vi "Set Security Level CORE.vi"(8 "error in (no error)":errorcluster, 9 "Set or Clear":T1, 10 "New Level":T2, 11 "Threat Deterent in":refnum<class "Threat Deterent.lvclass">) -> (0 "error out":errorcluster, 2 "Last Action Performed":string, 3 "Threat Deterent out":refnum<class "Threat Deterent.lvclass">)   [LabVIEW 2014, in "Threat Deterent.lvclass"]
uses:
  Threat Deterent.lvclass
  Security System/Security Level.ctl
  Security System/Set or Clear.ctl
  Threat Deterent.lvclass/Threat Deterent.ctl
  Electric Fence/Electric Fence.lvclass
  Security System/Security System.lvclass
  Rabbit Squad/Rabbit Squad.lvclass
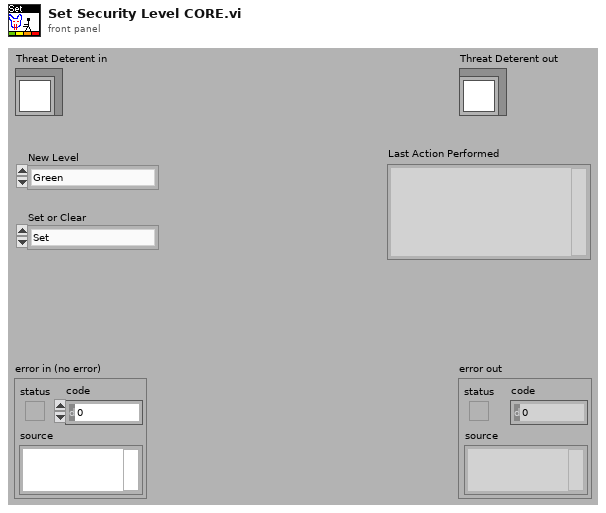
[diagram p1: front panel]
types:
  T1 = typedef "Security System.lvclass/Set or Clear.ctl" = enum16{"Set", "Clear"}
  T2 = typedef "Security System.lvclass/Security Level.ctl" = enum16{"Green", "Yellow", "Orange", "Red"}
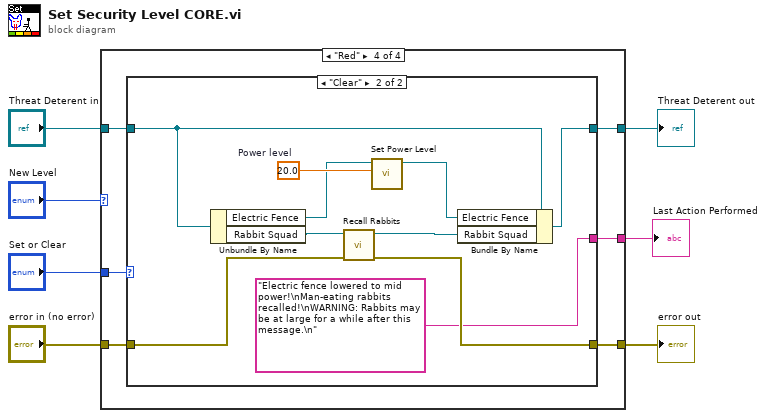
[diagram p0: block diagram]
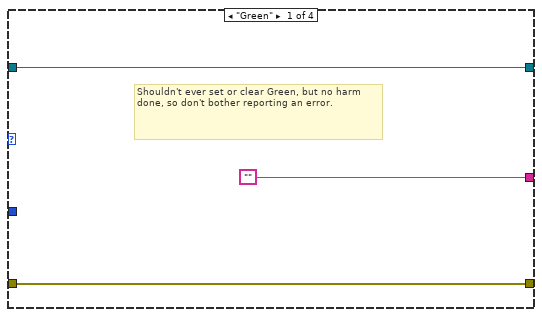
[diagram p2: hidden frame]
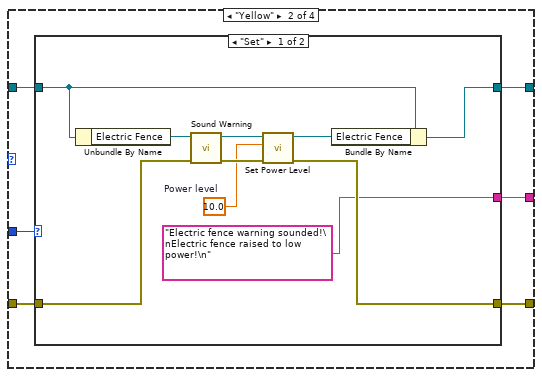
[diagram p3: hidden frame]
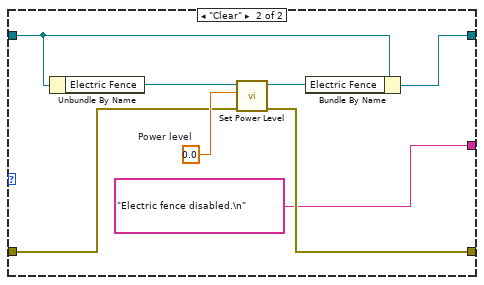
[diagram p4: hidden frame]
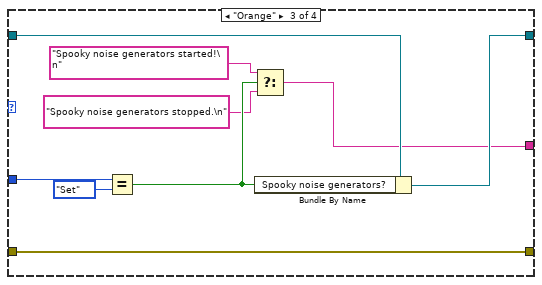
[diagram p5: hidden frame]
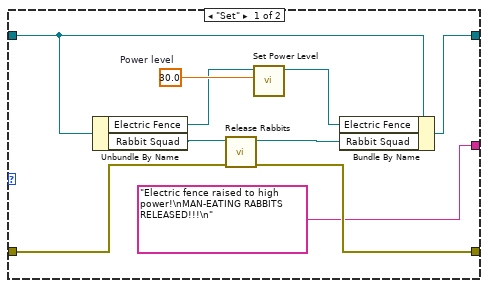
[diagram p6: hidden frame]
diagram:
  n1 = case shown="\"Red\"" "New Level" {
    tunnel: [w9 w12 w40 w45] -> w2
    tunnel: "Threat Deterent in" -> [w9 w13 w39 w46]
    tunnel: [w10 w15 w43 w48] -> w5
    tunnel: "error in (no error)" -> [w10 w14 w43 w47]
    tunnel: "Set or Clear" -> [_ w16 w42 w49]
    tunnel: ["" w11 w35 w44] -> w1
    frame "Green" {
      # "Shouldn't ever set or clear Green, but no harm done, so don't bother reporting an error."
    }
    frame "Yellow" {
      n2 = case shown="\"Set\"" w16 {
        tunnel: [w18 w28] -> w15
        tunnel: w14 -> [w19 w29]
        tunnel: w13 -> [w21 w32]
        tunnel: [w20 w31] -> w12
        tunnel: ["Electric fence warning sounded!\nElectric fence raised to low power!\n" ("Last Action Performed") "Electric fence disabled.\n" ("Last Action Performed")] -> w11
        frame "Set" {
          w23 = 10.0  # Power level
          n3 = Unbundle By Name(w21) -> ("Electric Fence"=w26:refnum<class "Electric Fence.lvclass">)
          n4 = call "Sound Warning.vi"("error in (no error)"=w19, "Electric Fence in"=w26) -> ("error out"=w24:errorcluster, "Electric Fence out"=w25:refnum<class "Electric Fence.lvclass">)  [unwired: 8 in]
          n5 = call "Set Power Level.vi"("error in (no error)"=w24, "Power level"=w23, "Electric Fence.lvclass in"=w25) -> ("error out"=w18:errorcluster, "Electric Fence.lvclass out"=w22:refnum<class "Electric Fence.lvclass">)  [unwired: 7 in]
          n6 = Bundle By Name(cluster=w21, "Electric Fence"=w22) -> (w20:refnum<class "Threat Deterent.lvclass">)
        }
        frame "Clear" {
          w34 = 0.0  # Power level
          n7 = Unbundle By Name(w32) -> ("Electric Fence"=w30:refnum<class "Electric Fence.lvclass">)
          n8 = call "Set Power Level.vi"("error in (no error)"=w29, "Power level"=w34, "Electric Fence.lvclass in"=w30) -> ("error out"=w28:errorcluster, "Electric Fence.lvclass out"=w33:refnum<class "Electric Fence.lvclass">)  [unwired: 7 in]
          n9 = Bundle By Name(cluster=w32, "Electric Fence"=w33) -> (w31:refnum<class "Threat Deterent.lvclass">)
        }
      }
    }
    frame "Orange" {
      n10 = Equal?(x=w42, y=Set_or_Clear."Set") -> (x = y?=w38:bool)
      n11 = Select(t="Spooky noise generators started!\n", s=w38, f="Spooky noise generators stopped.\n") -> (s? t:f=w35:string)
      n12 = Bundle By Name(cluster=w39, "Spooky noise generators?"=w38) -> (w40:refnum<class "Threat Deterent.lvclass">)
    }
    frame "Red" {
      n13 = case shown="\"Clear\"" w49 {
        tunnel: [w57 w67] -> w48
        tunnel: w47 -> [w58 w68]
        tunnel: w46 -> [w56 w66]
        tunnel: [w55 w65] -> w45
        tunnel: ["Electric fence raised to high power!\nMAN-EATING RABBITS RELEASED!!!\n" ("Last Action Performed") "Electric fence lowered to mid power!\nMan-eating rabbits recalled!\nWARNING: Rabbits may be at large for a while after this message.\n" ("Last Action Performed")] -> w44
        frame "Set" {
          w53 = 30.0  # Power level
          n14 = Unbundle By Name(w56) -> ("Electric Fence"=w52:refnum<class "Electric Fence.lvclass">, "Rabbit Squad"=w59:refnum<class "Rabbit Squad.lvclass">)
          n15 = call "Release Rabbits.vi"("error in (no error)"=w58, "Rabbit Squad in"=w59) -> ("error out"=w57:errorcluster, "Rabbit Squad out"=w54:refnum<class "Rabbit Squad.lvclass">)  [unwired: 8 in]
          n16 = call "Set Power Level.vi"("Power level"=w53, "Electric Fence.lvclass in"=w52) -> ("Electric Fence.lvclass out"=w51:refnum<class "Electric Fence.lvclass">)  [unwired: 8 in, 1 out]
          n17 = Bundle By Name(cluster=w56, "Electric Fence"=w51, "Rabbit Squad"=w54) -> (w55:refnum<class "Threat Deterent.lvclass">)
        }
        frame "Clear" {
          w63 = 20.0  # Power level
          n18 = Unbundle By Name(w66) -> ("Electric Fence"=w62:refnum<class "Electric Fence.lvclass">, "Rabbit Squad"=w69:refnum<class "Rabbit Squad.lvclass">)
          n19 = call "Recall Rabbits.vi"("error in (no error)"=w68, "Rabbit Squad in"=w69) -> ("error out"=w67:errorcluster, "Rabbit Squad out"=w64:refnum<class "Rabbit Squad.lvclass">)  [unwired: 8 in]
          n20 = call "Set Power Level.vi"("Power level"=w63, "Electric Fence.lvclass in"=w62) -> ("Electric Fence.lvclass out"=w61:refnum<class "Electric Fence.lvclass">)  [unwired: 8 in, 1 out]
          n21 = Bundle By Name(cluster=w66, "Electric Fence"=w61, "Rabbit Squad"=w64) -> (w65:refnum<class "Threat Deterent.lvclass">)
        }
      }
    }
  }
  "error out" <- w5
  "Threat Deterent out" <- w2
  "Last Action Performed" <- w1
